vi "Set Children Symbols.vi"(8 "error in":errorcluster, 10 "Parent tag":refnum<class "Tree Tag Class.lvclass">, 11 "Tree_LVOOP in":refnum<class "Tree Class.lvclass">) -> (0 "error out":errorcluster, 3 "Tree_LVOOP out":refnum<class "Tree Class.lvclass">)   [LabVIEW 2012, in "Tree Tools.lvlib" / "Tree Class.lvclass"]
uses:
  Tree Class.lvclass
  Tree Tag Class/Tree Tag Class.lvclass
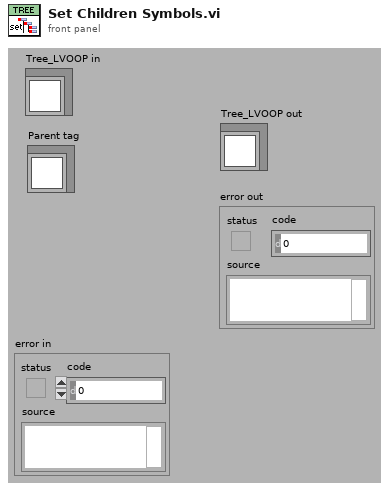
[diagram p1: front panel]
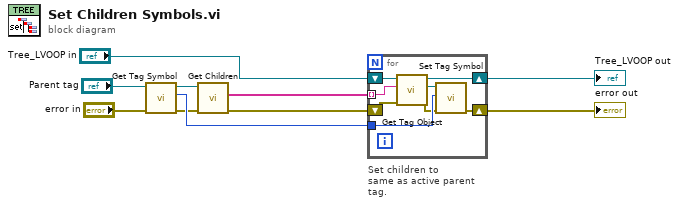
[diagram p0: block diagram]
diagram:
  # "Set children to\nsame as active parent\ntag."
  n1 = call-dynamic "Get Tag Symbol.vi"("error in (no error)"="error in", "Tag_LVOOP in"="Parent tag") -> ("error out"=w2:errorcluster, "Symbol Index"=w3:i32, "Tag_LVOOP out"=w4:refnum<class "Tree Tag Class.lvclass">)  [unwired: 7 in]
  n2 = call-dynamic "Get Children.vi"("error in (no error)"=w2, "Tag_LVOOP in"=w4) -> ("error out"=w9:errorcluster, "Children Tag Strings"=w7:string[])  [unwired: 6 in, 2 out]
  n3 = for {
    tunnel: w7 -> [w17] mode=indexing
    tunnel: w3 -> [w15]
    shift-right: [w14] -> w8
    shift-left: "Tree_LVOOP in" -> [w18]
    shift-right: [w11] -> w10
    shift-left: w9 -> [w13]
    n4 = call-dynamic "Get Tag Object.vi"("error in (no error)"=w13, "Tag (string)"=w17, "Tree_LVOOP in"=w18) -> ("error out"=w12:errorcluster, "Tag"=w16:refnum<class "Tree Tag Class.lvclass">, "Tree_LVOOP out"=w14:refnum<class "Tree Class.lvclass">)  [unwired: 1 in, 5 out]
    n5 = call-dynamic "Set Tag Symbol.vi"("error in (no error)"=w12, "Symbol Index"=w15, "Tag_LVOOP in"=w16) -> ("error out"=w11:errorcluster)  [unwired: 7 in, 1 out]
  }
  "error out" <- w10
  "Tree_LVOOP out" <- w8
